vi "Button_Click.vi"(0 "Button_1":bool caption="Button 1", 5 "Button_2":bool caption="Button 2", 11 "Error_In":errorcluster) -> (15 "Error_Out":errorcluster)   [LabVIEW 2023]
doc: "This VI alternatively Clicks two boolean buttons until key down happens,"
uses:
  Controls/Click_On.ctl
panel:
  out "Button_2_Indicator":bool caption="Button 2 Indicator"
  out "Button_1_Indicator":bool caption="Button 1 Indicator"
  # "."
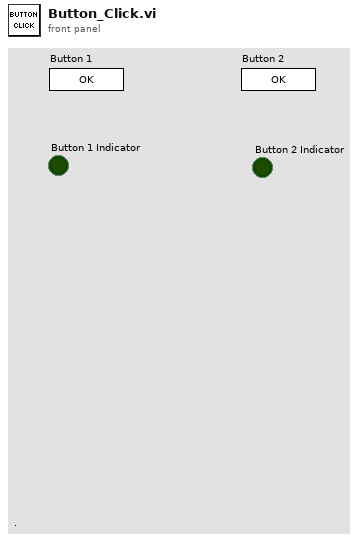
[diagram p1: front panel]
types:
  T1 = typedef "Click_On.ctl" = enum16{"Button 1", "Button 2"}
  T2 = typedef "LVRectTypeDef.ctl" = cluster{"Left":i16, "Top":i16, "Right":i16, "Bottom":i16}
  T3 = typedef "LVPositionTypeDef.ctl" = cluster{"Left":i32, "Top":i32}
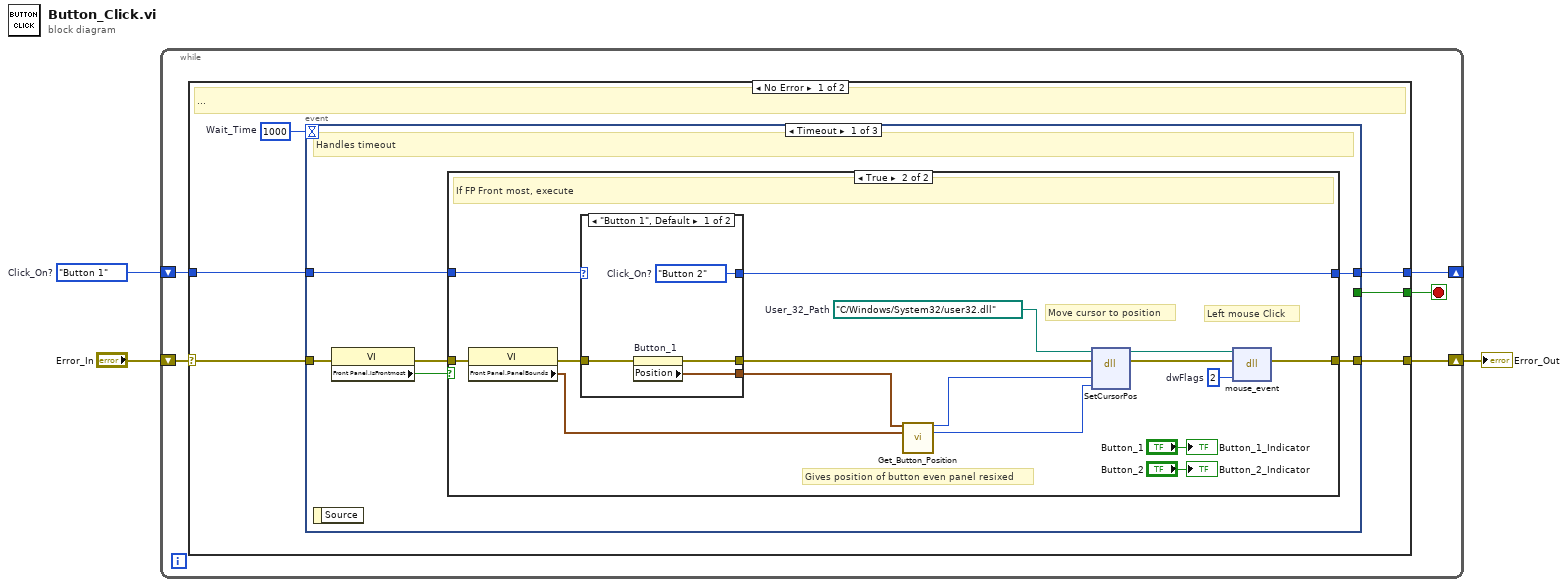
[diagram p0: block diagram]
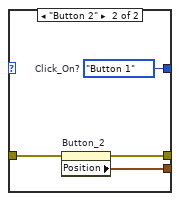
[diagram p3: hidden frame]
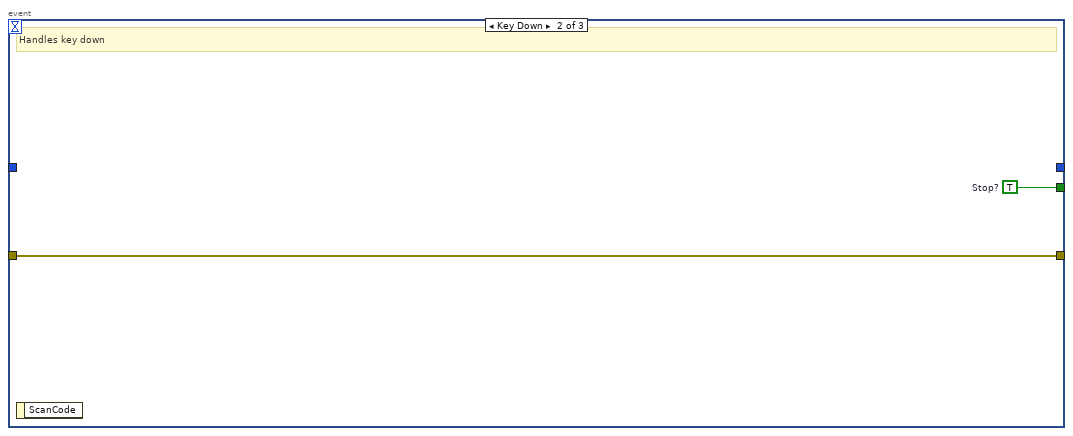
[diagram p4: hidden frame]
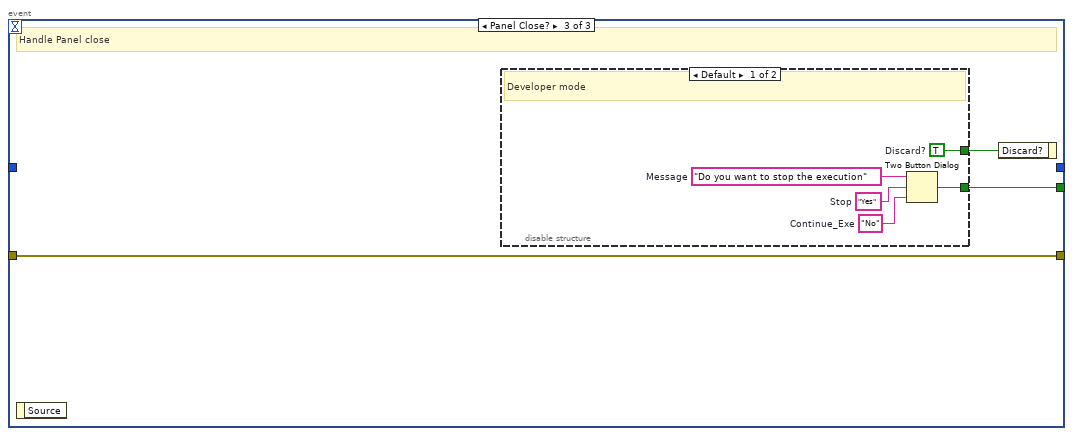
[diagram p5: hidden frame]
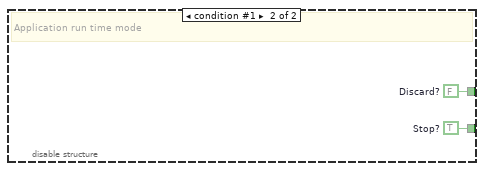
[diagram p6: hidden frame]
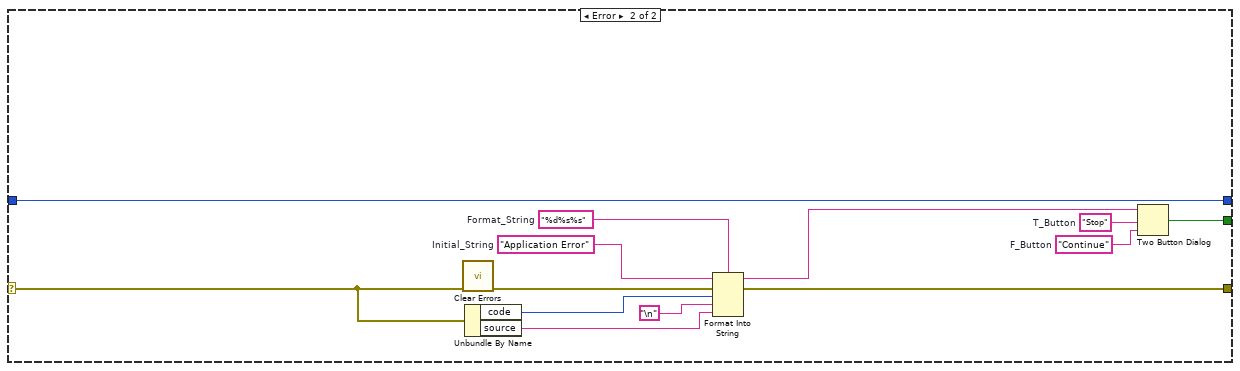
[diagram p7: hidden frame]
diagram:
  w2 = Click_On."Button 1"  # Click_On?
  n1 = while {
    shift-right: [w7] -> _
    shift-left: w2 -> [w5]
    shift-right: [w6] -> w3
    shift-left: "Error_In" -> [w8]
    stop <- w4 stop-if-true
    n2 = case shown="No Error" w8 {
      selector: w8 -> [w13 w59]
      tunnel: [w12 w60] -> w7
      tunnel: [w11 w62] -> w6
      tunnel: w5 -> [w10 w60]
      tunnel: [w9 w61] -> w4
      frame No Error {
        w14 = 1000  # Wait_Time
        # "..."
        n3 = event shown="[0] Timeout" {
          selector: _ -> [_ _ _]
          dyn-events: _ -> [_ _ _]
          timeout: w14 -> [_ _ _]
          tunnel: w13 -> [w17 w48 w51]
          tunnel: [w20 _ _] -> w12
          tunnel: [w18 w48 w51] -> w11
          tunnel: w10 -> [w19 _ _]
          tunnel: [_ w47 w50] -> w9
          event Timeout {
            # "Handles timeout"
            n4 = event-data() -> ()  [unwired: 1 in, 1 out]
            n5 = property class="VI"(error in=w17) -> (error out=w16:errorcluster, "Front Panel.IsFrontmost"=w15:bool)  [unwired: 1 in, 1 out]
            n6 = case shown="True" w15 {
              tunnel: [w21 w38] -> w20
              tunnel: w19 -> [w21 w37]
              tunnel: [w22 w35] -> w18
              tunnel: w16 -> [w22 w29]
              frame False {
                # "If FP not front most, dont execute"
              }
              frame True {
                w26 = path "C:/Windows/System32/user32.dll"  # User_32_Path
                w34 = 2  # dwFlags
                # "Gives position of button even panel resixed"
                # "Left mouse Click"
                # "Move cursor to position"
                # "If FP Front most, execute"
                n7 = property class="VI"(error in=w29) -> (error out=w28:errorcluster, "Front Panel.PanelBounds"=w27:T2)  [unwired: 1 in, 1 out]
                n8 = case shown="\"Button 1\", Default" w37 {
                  tunnel: w28 -> [w42 w44]
                  tunnel: [w41 w46] -> w31
                  tunnel: [w40 w45] -> w30
                  tunnel: [w39 w43] -> w38
                  frame "Button 1", Default {
                    w39 = Click_On."Button 2"  # Click_On?
                    n9 = property on="Button_1" class="Bool (strict)"(error in=w42) -> (error out=w41:errorcluster, "Position"=w40:T3)  [unwired: 1 in, 1 out]
                  }
                  frame "Button 2" {
                    w43 = Click_On."Button 1"  # Click_On?
                    n10 = property on="Button_2" class="Bool (strict)"(error in=w44) -> (error out=w46:errorcluster, "Position"=w45:T3)  [unwired: 1 in, 1 out]
                  }
                }
                n11 = call "Get_Button_Position.vi"("Position"=w30, "FP_Bounds"=w27) -> ("Left"=w32:i32, "Top"=w33:i32)  [unwired: 12 in]
                n12 = dll-call lib="?" fn="SetCursorPos"(path in=w26, error in=w31, "X_Coord"=w32, "Y_Coord"=w33) -> (path out=w25:path, error out=w36:errorcluster)  [unwired: 4 in]
                n13 = dll-call lib="?" fn="mouse_event"(path in=w25, error in=w36, "dwFlags"=w34) -> (error out=w35:errorcluster)  [unwired: 3 in, 1 out]
                "Button_1_Indicator" <- "Button_1"
                "Button_2_Indicator" <- "Button_2"
              }
            }
          }
          event Key Down {
            w47 = TRUE  # Stop?
            # "Handles key down"
            n14 = event-data() -> ()  [unwired: 1 in, 1 out]
          }
          event Panel Close? {
            # "Handle Panel close"
            n15 = event-data() -> ()  [unwired: 1 in, 1 out]
            n16 = disable-structure shown="Default" {
              disable-tunnel: [w53 w57] -> w50
              disable-tunnel: [w52 w58] -> w49
              frame condition #0 (active) {
                w52 = TRUE  # Discard?
                w54 = "No"  # Continue_Exe
                w55 = "Yes"  # Stop
                w56 = "Do you want to stop the execution"  # Message
                # "Developer mode"
                n17 = Two Button Dialog(message=w56, 1:w54, 2:w55) -> (T button?=w53:bool)
              }
              frame condition #1 {
                w57 = TRUE  # Stop?
                w58 = FALSE  # Discard?
                # "Application run time mode"
              }
            }
            n18 = event-data("Discard?"=w49) -> ()  [unwired: 1 in, 1 out]
          }
        }
      }
      frame Error {
        w67 = "%d%s%s"  # Format_String
        w68 = "Application Error"  # Initial_String
        w69 = "Stop"  # T_Button
        w70 = "Continue"  # F_Button
        n19 = call <vilib>:"Clear Errors.vi"("error in (no error)"=w59) -> ("error out"=w65:errorcluster)  [unwired: 5 in, 1 out]
        n20 = Unbundle By Name(w59) -> ("code"=w64:i32, "source"=w63:string)
        n21 = Format Into String(format string=w67, initial string=w68, error in=w65, w64, "\n", w63) -> (resulting string=w71:string, error out=w62:errorcluster)
        n22 = Two Button Dialog(message=w71, 1:w70, 2:w69) -> (T button?=w61:bool)
      }
    }
  }
  "Error_Out" <- w3
